vi "binsearch.vi"(9 "String":string, 10 "indices":i32[](array[numeric]), 11 "strings":string[](array[string])) -> (3 "index":i32)   [LabVIEW 2013]
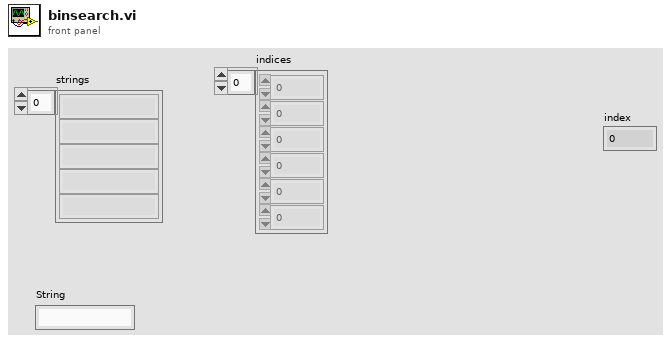
[diagram p1: front panel]
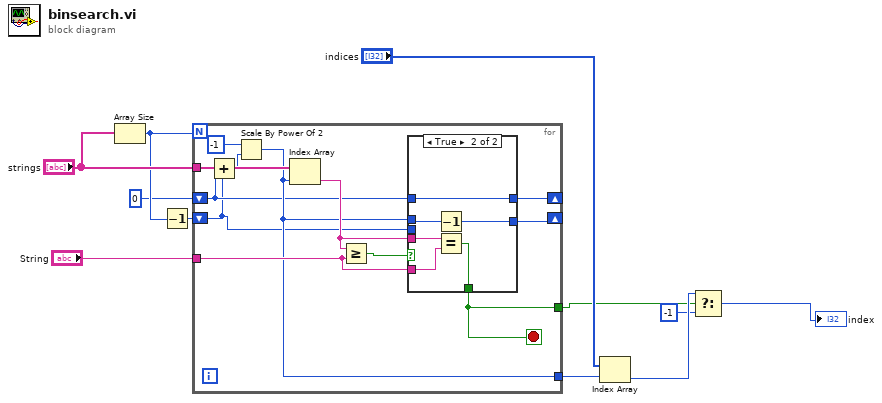
[diagram p0: block diagram]
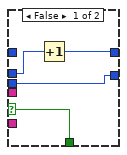
[diagram p2: hidden frame]
diagram:
  n1 = Array Size(array="strings") -> (size(s)=w9:i32)
  n2 = Decrement(x=w9) -> (x-1=w1:i32)
  n3 = for {
    N: w9 -> [_]
    tunnel: "strings" -> [w23]
    tunnel: "String" -> [w19]
    shift-right: [w15] -> _
    shift-left: w1 -> [w12]
    shift-right: [w13] -> _
    shift-left: 0 -> [w14]
    tunnel: [w18] -> w4
    tunnel: [w16] -> w7
    stop <- w18 stop-if-true
    n4 = Add(x=w14, y=w12) -> (x+y=w21:i32)
    n5 = Scale By Power Of 2(n=i16 -1, x=w21) -> (x*2^n=w16:i32)
    n6 = Index Array(array=w23, index=w16) -> (element=w20:string)
    n7 = Greater Or Equal?(x=w20, y=w19) -> (x >= y?=w17:bool)
    n8 = case shown="True" w17 {
      selector: w17 -> [w27 _]
      tunnel: w20 -> [_ w33]
      tunnel: w19 -> [_ w32]
      tunnel: [w27 w31] -> w18
      tunnel: w16 -> [w26 w30]
      tunnel: [w25 w29] -> w15
      tunnel: w14 -> [_ w28]
      tunnel: [w24 w28] -> w13
      tunnel: w12 -> [w25 _]
      frame False {
        n9 = Increment(x=w26) -> (x+1=w24:i32)
      }
      frame True {
        n10 = Decrement(x=w30) -> (x-1=w29:i32)
        n11 = Equal?(x=w33, y=w32) -> (x = y?=w31:bool)
      }
    }
  }
  n12 = Index Array(array="indices", index=w7) -> (element=w5:i32)
  n13 = Select(t=w5, s=w4, f=-1) -> (s? t:f=→"index":i32)
